vi "DT_Triangle Manager_Get Adj Point_by Edge.vi"(8 "point idx 2":i32, 9 "point idx 1":i32, 10 "triangle":i32, 11 "Triangles In":i32[][](array[numeric])) -> (1 "adj point idx":i32, 2 "adj triangle":i32)   [LabVIEW 2017, in "NI_AAL_Geometry.lvlib"]
uses:
  <vilib>/Analysis/NI_AAL_Geometry.lvlib
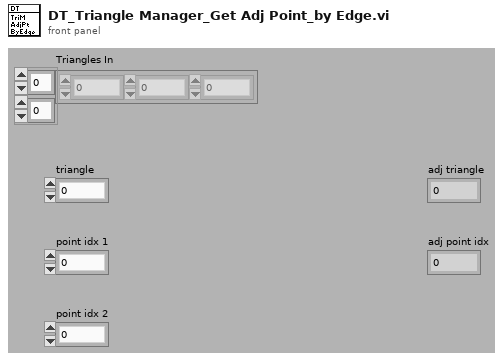
[diagram p1: front panel]
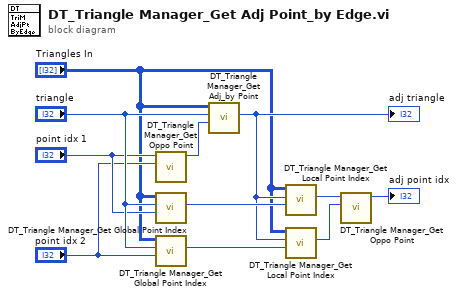
[diagram p0: block diagram]
diagram:
  n1 = call <vilib>:"DT_Triangle Manager_Get Oppo Point.vi"("point idx 2"="point idx 2", "point idx 1"="point idx 1") -> ("oppo point idx"=w11:i32)  [unwired: 9 out]
  n2 = call <vilib>:"DT_Triangle Manager_Get Global Point Index.vi"("local idx"="point idx 1", "triangle"="triangle", "Triangles"="Triangles In") -> ("global idx"=w7:i32)  [unwired: 8 out]
  n3 = call <vilib>:"DT_Triangle Manager_Get Global Point Index.vi"("local idx"="point idx 2", "triangle"="triangle", "Triangles"="Triangles In") -> ("global idx"=w5:i32)  [unwired: 8 out]
  n4 = call <vilib>:"DT_Triangle Manager_Get Adj_by Point.vi"("point idx"=w11, "triangle"="triangle", "Triangles In"="Triangles In") -> ("adj triangle"=w6:i32)  [unwired: 8 out]
  "adj triangle" <- w6
  n5 = call <vilib>:"DT_Triangle Manager_Get Local Point Index.vi"("global idx"=w7, "triangle"=w6, "Triangles"="Triangles In") -> ("local idx"=w4:i32)  [unwired: 8 out]
  n6 = call <vilib>:"DT_Triangle Manager_Get Local Point Index.vi"("global idx"=w5, "triangle"=w6, "Triangles"="Triangles In") -> ("local idx"=w3:i32)  [unwired: 8 out]
  n7 = call <vilib>:"DT_Triangle Manager_Get Oppo Point.vi"("point idx 2"=w3, "point idx 1"=w4) -> ("oppo point idx"=→"adj point idx":i32)  [unwired: 9 out]
